vi "HRM-Stage4-Hardware_daqmx_main.vi"(8 "error in (no error)":errorcluster, 11 "Init cluster":T1) -> (0 "error out":errorcluster)   [LabVIEW 2020]
uses:
  initclose/HRM-Stage4-init_cluster.ctl
  initclose/HRM-Stage4-User_events.ctl
panel:
  in  "Aqn?":bool
  in  "stop":bool
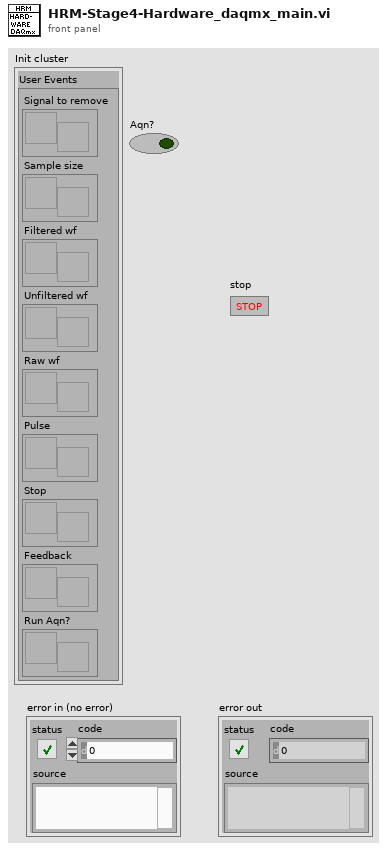
[diagram p1: front panel]
types:
  T1 = typedef "HRM-Stage4-init_cluster.ctl" = cluster{"User Events":T2}
  T2 = typedef "HRM-Stage4-User_events.ctl" = cluster{"Signal to remove":refnum<user-event>, "Sample size":refnum<user-event>, "Filtered wf":refnum<user-event>, "Unfiltered wf":refnum<user-event>, "Raw wf":refnum<user-event>, "Pulse":refnum<user-event>, "Stop":refnum<user-event>, "Feedback":refnum<user-event>, "Run Aqn?":refnum<user-event>}
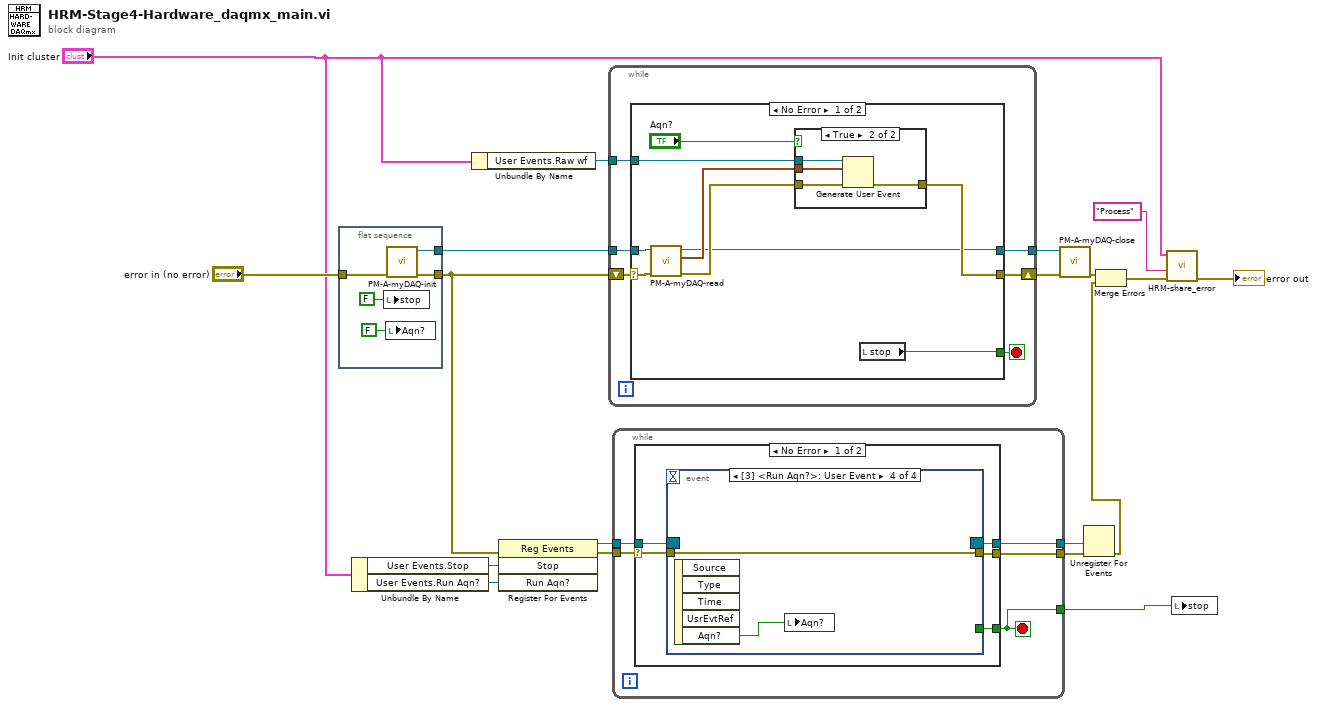
[diagram p0: block diagram]
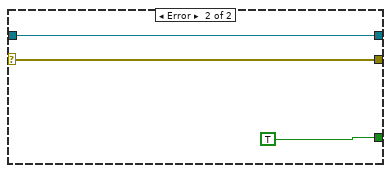
[diagram p3: hidden frame]
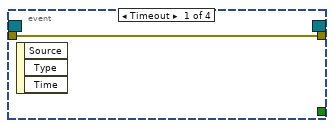
[diagram p4: hidden frame]
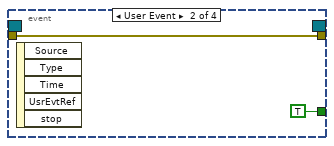
[diagram p5: hidden frame]
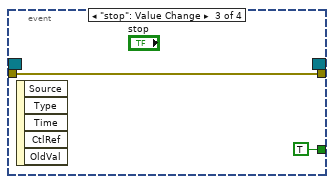
[diagram p6: hidden frame]
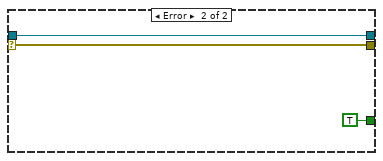
[diagram p7: hidden frame]
diagram:
  n1 = flat-sequence {
    tunnel: "error in (no error)" -> [w24]
    tunnel: [w23] -> w10
    tunnel: [w21] -> w7
    frame #0 {
      n2 = local write "stop"(FALSE ("stop")) -> ()
      n3 = local write "Aqn?"(FALSE ("Aqn?")) -> ()
      n4 = call "PM-A-myDAQ-init.vi"("error in"=w24) -> ("error out"=w21:errorcluster, "Refnum out"=w23:refnum<k21>)  [unwired: 9 in]
    }
  }
  n5 = Unbundle By Name("Init cluster") -> ("User Events.Stop"=w13:refnum<user-event>, "User Events.Run Aqn?"=w1:refnum<user-event>)
  n6 = Unbundle By Name("Init cluster") -> ("User Events.Raw wf"=w11:refnum<user-event>)
  n7 = register-events(error in=w7, w13, w1) -> (reference out=w15:refnum<event-registration>, error out=w12:errorcluster)  [unwired: 1 in]
  n8 = while {
    tunnel: w10 -> [w30]
    tunnel: [w28] -> w9
    shift-right: [w27] -> w8
    shift-left: w7 -> [w29]
    tunnel: w11 -> [w25]
    stop <- w26 stop-if-true
    n9 = case shown="No Error" w29 {
      selector: w29 -> [w35 w46]
      tunnel: w30 -> [w34 w45]
      tunnel: [w31 w45] -> w28
      tunnel: [w39 w46] -> w27
      tunnel: [w37 TRUE ("Stop")] -> w26
      tunnel: w25 -> [w38 _]
      frame No Error {
        n10 = call "PM-A-myDAQ-read.vi"("error in (no error)"=w35, "Refnum in"=w34) -> ("error out"=w33:errorcluster, "data"=w32:waveform(dbl), "Refnum out"=w31:refnum<k21>)  [unwired: 7 in]
        n11 = case shown="True" "Aqn?" {
          tunnel: [w40 w44] -> w39
          tunnel: w38 -> [_ w43]
          tunnel: w33 -> [w40 w42]
          tunnel: w32 -> [_ w41]
          frame False {
          }
          frame True {
            n12 = Generate User Event(user event=w43, event data cluster=w41, error in=w42) -> (error out=w44:errorcluster)  [unwired: 1 in, 1 out]
          }
        }
        n13 = local read "stop"() -> (w37:bool)
      }
      frame Error {
      }
    }
  }
  n14 = while {
    tunnel: w12 -> [w52]
    tunnel: w15 -> [w51]
    tunnel: [w50] -> w16
    tunnel: [w49] -> w17
    tunnel: [w48] -> w6
    stop <- w48 stop-if-true
    n15 = case shown="No Error" w52 {
      selector: w52 -> [w55 w66]
      tunnel: w51 -> [w57 w65]
      tunnel: [w56 TRUE] -> w48
      tunnel: [w54 w66] -> w49
      tunnel: [w53 w65] -> w50
      frame No Error {
        n16 = event shown="[3] <Run Aqn?>: User Event" {
          selector: w57 -> [_ _ _ _]
          dyn-events: [_ _ _ _] -> w53
          timeout: _ -> [_ _ _ _]
          tunnel: [_ TRUE TRUE _] -> w56
          tunnel: w55 -> [w58 w59 w62 w64]
          tunnel: [w58 w59 w62 w64] -> w54
          event Timeout {
            n17 = event-data() -> ()  [unwired: 1 in, 3 out]
          }
          event User Event {
            n18 = event-data() -> ()  [unwired: 1 in, 5 out]
          }
          event "stop": Value Change {
            n19 = event-data() -> ()  [unwired: 1 in, 5 out]
          }
          event User Event {
            n20 = event-data() -> ("Aqn?"=w63:bool)  [unwired: 1 in, 4 out]
            n21 = local write "Aqn?"(w63) -> ()
          }
        }
      }
      frame Error {
      }
    }
  }
  n22 = call "PM-A-myDAQ-close.vi"("error in (no error)"=w8, "Refnum in"=w9) -> ("error out"=w18:errorcluster)  [unwired: 9 in]
  n23 = Unregister For Events(event registration refnum=w16, error in=w17) -> (error out=w19:errorcluster)
  n24 = Merge Errors(w18, w19) -> (w4:errorcluster)
  n25 = call "HRM-share_error.vi"("error in (no error)"=w4, "module name"="Process", "Init cluster"="Init cluster") -> ("error out"=→"error out":errorcluster)  [unwired: 8 in]
  n26 = local write "stop"(w6) -> ()
